vi "anna_results.vi"() -> ()   [LabVIEW 2009]
uses:
  <vilib>/Analysis/NI_AALPro.lvlib
panel:
  out "total spots":i32
  in  "add this file":bool
  out "All Files":path[](array[path])
  in  "clear xy":bool
  in  "store xy":bool
  out "XY Graph 2":cluster{"selected":dbl[], "selected":dbl[]}[](graph)
  in  "clear hist":bool
  in  "store hist":bool
  out "Histogram Graph 2":T1(graph)
  in  "export":bool
  in  "stop":bool
  in  "plot":bool
  out "selected":dbl[][](array[numeric])
  out "names":string[](array[string])
  out "XY Graph":cluster{"selected":dbl[], "selected":dbl[]}(graph)
  in  "plot y":u16(ring) items=["Spot No.", "plane", "Coordinates left", "Coordinates top", "Coordinates right", "Coordinates bottom", "TAC Window 1", "TAC Window 2", "Lifetime[ns] (sum)", "Lifetime[ns] (channel 1)", "Lifetime[ns] (channel 2)", "Lifetime[ns] (channel 3)", "tauerror (sum)", "tauerror (channel 1)", "tauerror (channel 2)", "tauerror (channel 3)", "F2-Value overall", "overall intensity (sum)", "overall intensity (channel 1)", "overall intensity (channel 2)", "overall intensity (channel 3)", "F2-Value TAC", "TAC intensity (sum)", "TAC intensity (channel 1)", "TAC intensity (channel 2)", "TAC intensity (channel 3)"]
  in  "plot x":u16(ring) items=["Spot No.", "plane", "Coordinates left", "Coordinates top", "Coordinates right", "Coordinates bottom", "TAC Window 1", "TAC Window 2", "Lifetime[ns] (sum)", "Lifetime[ns] (channel 1)", "Lifetime[ns] (channel 2)", "Lifetime[ns] (channel 3)", "tauerror (sum)", "tauerror (channel 1)", "tauerror (channel 2)", "tauerror (channel 3)", "F2-Value overall", "overall intensity (sum)", "overall intensity (channel 1)", "overall intensity (channel 2)", "overall intensity (channel 3)", "F2-Value TAC", "TAC intensity (sum)", "TAC intensity (channel 1)", "TAC intensity (channel 2)", "TAC intensity (channel 3)"]
  out "Histogram Graph":T2(graph)
  in  "# bins":i32
  in  "min":dbl format="%0.2f"
  in  "max":dbl format="%0.2f"
  in  "histogram":u16(ring) items=["Spot No.", "plane", "Coordinates left", "Coordinates top", "Coordinates right", "Coordinates bottom", "TAC Window 1", "TAC Window 2", "Lifetime[ns] (sum)", "Lifetime[ns] (channel 1)", "Lifetime[ns] (channel 2)", "Lifetime[ns] (channel 3)", "tauerror (sum)", "tauerror (channel 1)", "tauerror (channel 2)", "tauerror (channel 3)", "F2-Value overall", "overall intensity (sum)", "overall intensity (channel 1)", "overall intensity (channel 2)", "overall intensity (channel 3)", "F2-Value TAC", "TAC intensity (sum)", "TAC intensity (channel 1)", "TAC intensity (channel 2)", "TAC intensity (channel 3)"]
  in  "Selection":T3(array[cluster]) {"column" items=["Spot No.", "plane", "Coordinates left", "Coordinates top", "Coordinates right", "Coordinates bottom", "TAC Window 1", "TAC Window 2", "Lifetime[ns] (sum)", "Lifetime[ns] (channel 1)", "Lifetime[ns] (channel 2)", "Lifetime[ns] (channel 3)", "tauerror (sum)", "tauerror (channel 1)", "tauerror (channel 2)", "tauerror (channel 3)", "F2-Value overall", "overall intensity (sum)", "overall intensity (channel 1)", "overall intensity (channel 2)", "overall intensity (channel 3)", "F2-Value TAC", "TAC intensity (sum)", "TAC intensity (channel 1)", "TAC intensity (channel 2)", "TAC intensity (channel 3)"]}
  out "raw":dbl[][](array[numeric])
  in  "file (use dialog)":path
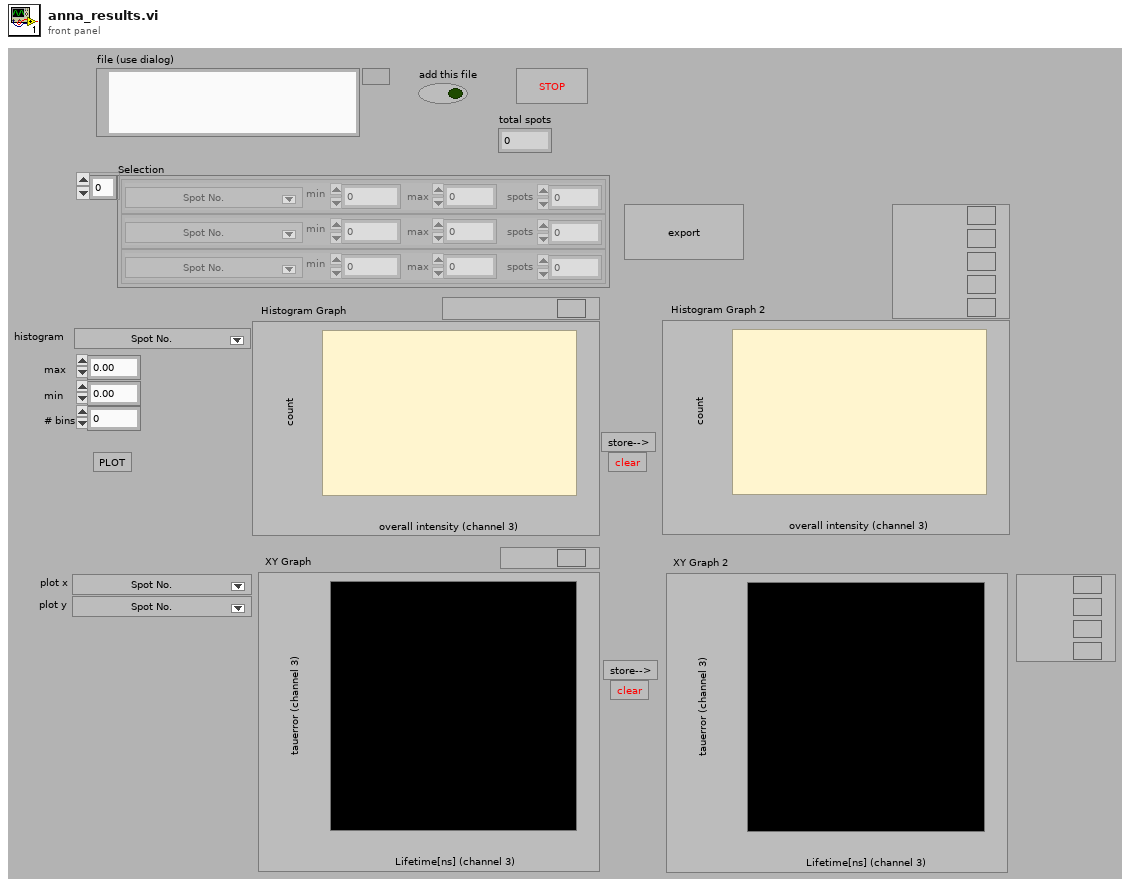
[diagram p1: front panel]
types:
  T1 = cluster{"X Values":dbl[], "Histogram: h(x)":i32[]}[]
  T2 = cluster{"X Values":dbl[], "Histogram: h(x)":i32[]}
  T3 = cluster{"column":u16, "min":dbl, "max":dbl, "spots ":i16}[]
  T4 = cluster{"column":u16, "min":dbl, "max":dbl, "spots ":i16}
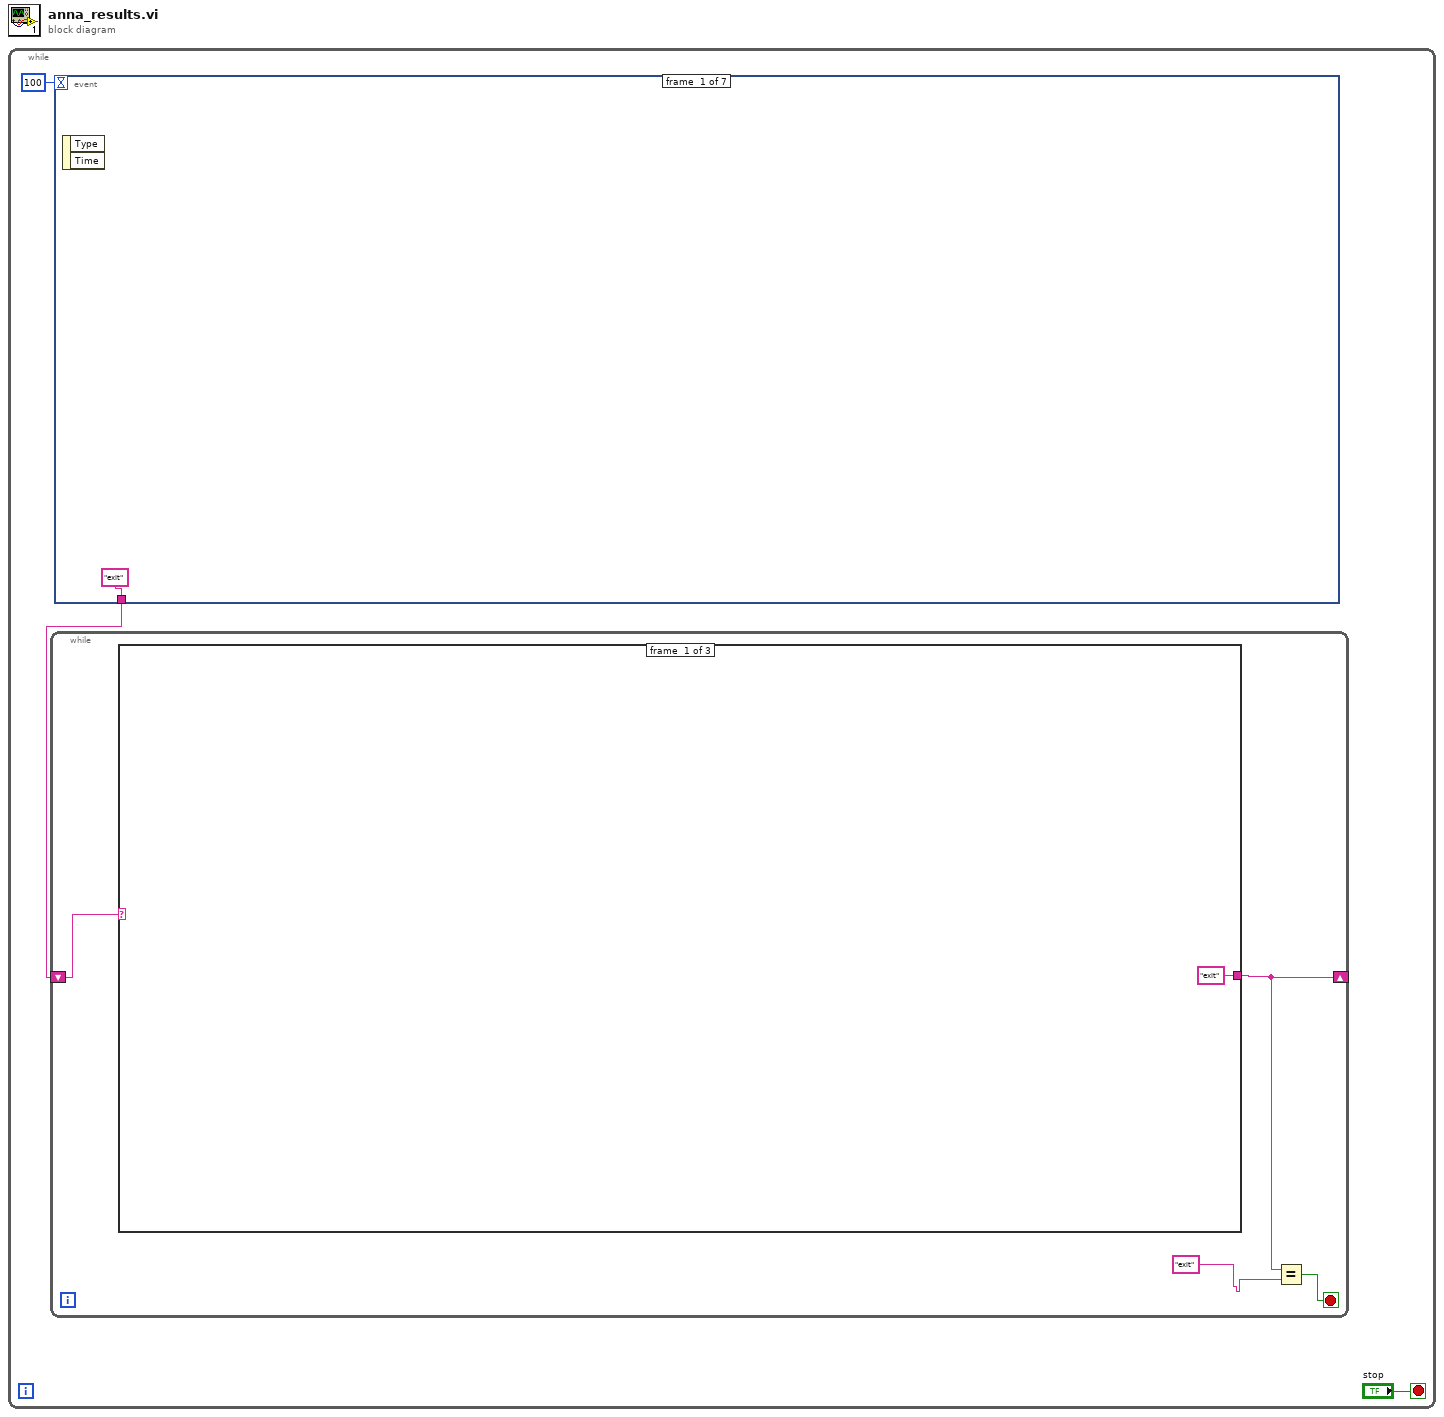
[diagram p0: block diagram]
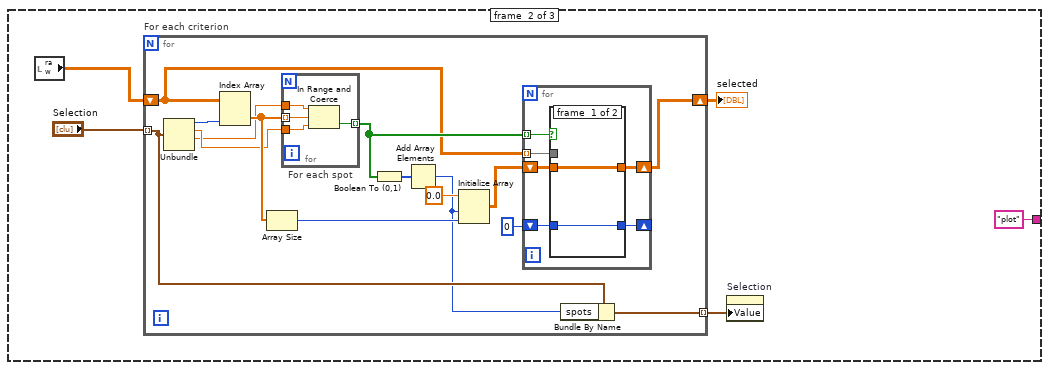
[diagram p2: hidden frame]
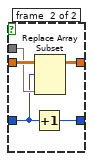
[diagram p3: hidden frame]
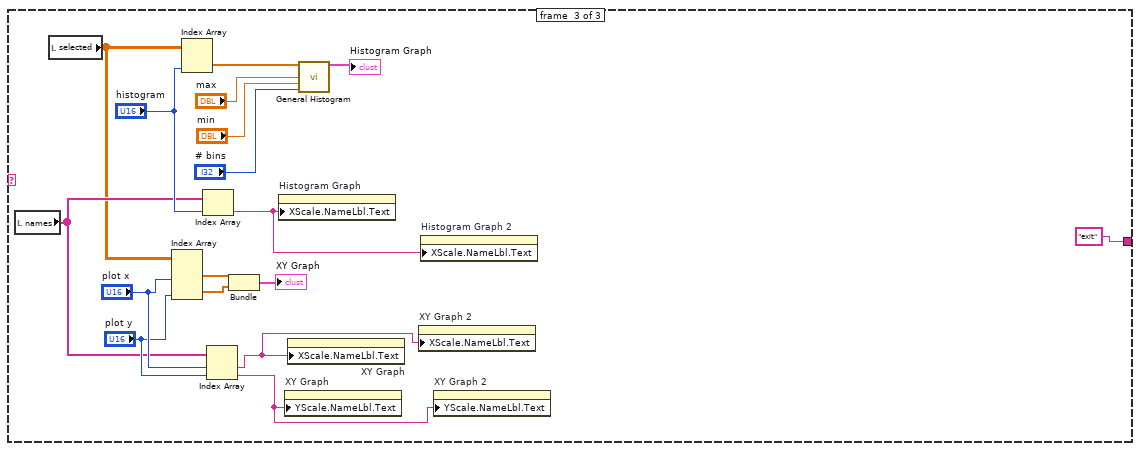
[diagram p4: hidden frame]
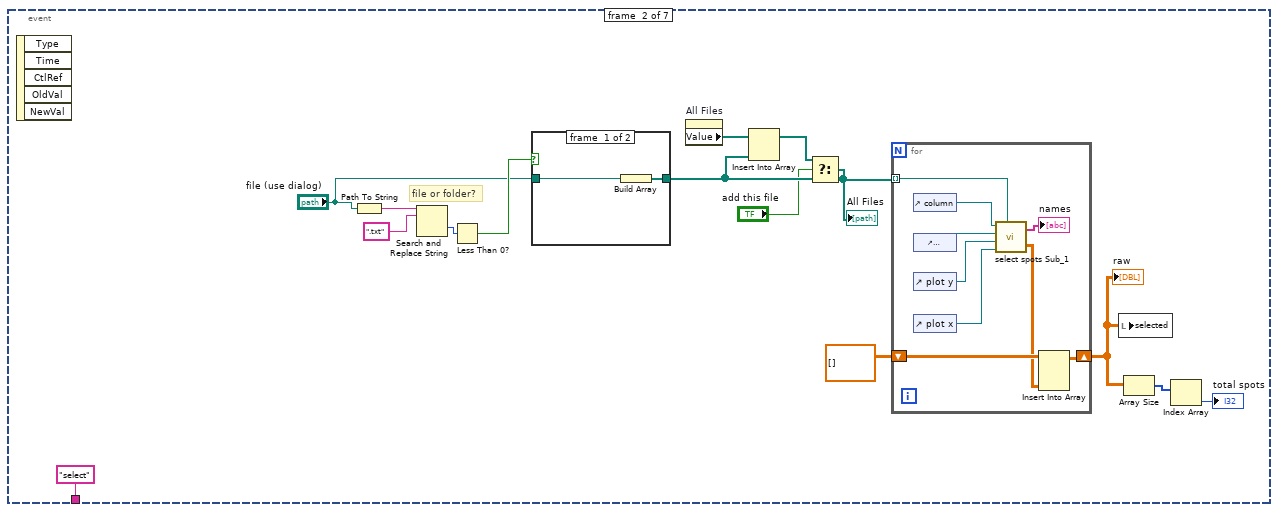
[diagram p5: hidden frame]
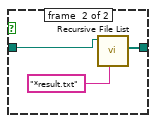
[diagram p6: hidden frame]
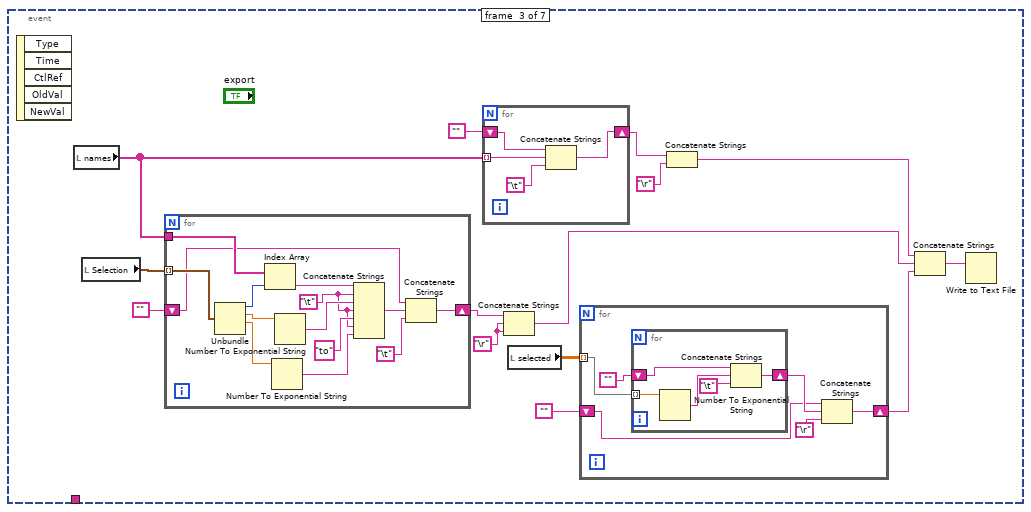
[diagram p7: hidden frame]
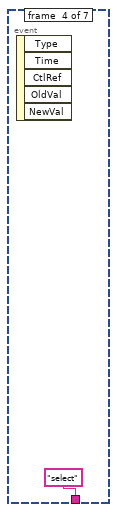
[diagram p8: hidden frame]
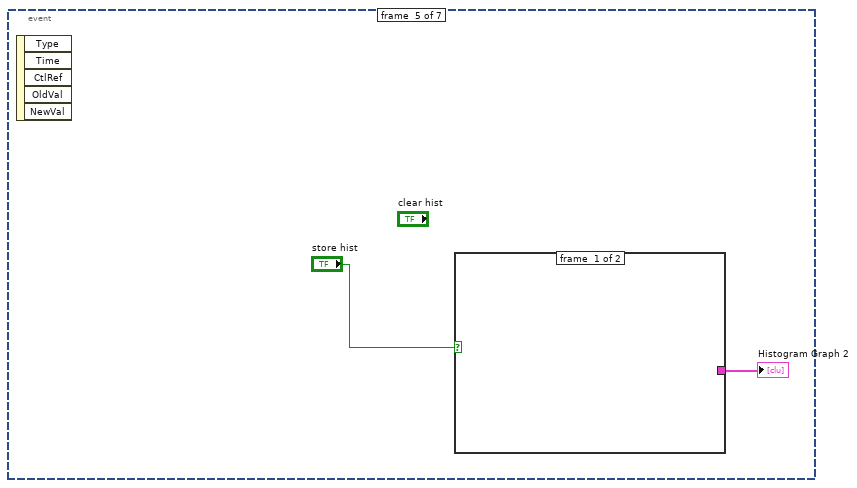
[diagram p9: hidden frame]
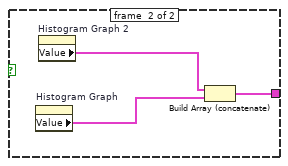
[diagram p10: hidden frame]
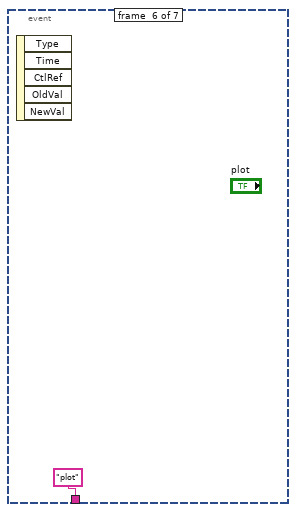
[diagram p11: hidden frame]
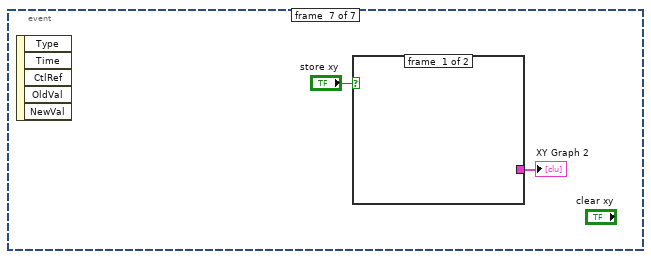
[diagram p12: hidden frame]
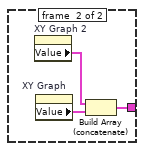
[diagram p13: hidden frame]
diagram:
  n1 = while {
    stop <- "stop" stop-if-true
    n2 = event shown="[1] \"file (use dialog)\": Value Change" {
      selector: _ -> [_ _ _ _ _ _ _]
      dyn-events: _ -> [_ _ _ _ _ _ _]
      timeout: 100 -> [_ _ _ _ _ _ _]
      tunnel: ["exit" "select" _ "select" _ "plot" _] -> w3
      event #0 {
        n3 = event-data() -> ()  [unwired: 1 in, 2 out]
      }
      event #1 {
        # "file or folder?"
        n4 = event-data() -> ()  [unwired: 1 in, 5 out]
        n5 = Path To String(path="file (use dialog)") -> (string=w76:string)
        n6 = Search and Replace String(input string=w76, search string=".txt") -> (offset past replacement=w74:i32)  [unwired: 6 in, 3 out]
        n7 = Less Than 0?(x=w74) -> (x < 0?=w73:bool)
        n8 = case shown="False" w73 {
          tunnel: [w79 w81] -> w69
          tunnel: "file (use dialog)" -> [w80 w83]
          frame #0 {
            n9 = Build Array(w80) -> (w79:path[])
          }
          frame #1 {
            n10 = call <vilib>:"Recursive File List.vi"("pattern"="*result.txt", "Folder Path"=w83) -> ("All Files in Dir"=w81:path[])  [unwired: 5 in, 4 out]
          }
        }
        n11 = property on="All Files" class="Arr (strict)"() -> ("Value"=w70:path[])  [unwired: 2 in, 2 out]
        n12 = Insert Into Array(array=w70, new element=w69) -> (w68:path[])  [unwired: 1 in]
        n13 = Select(t=w68, s="add this file", f=w69) -> (s? t:f=w71:path[])
        "All Files" <- w71
        n14 = for {
          tunnel: w71 -> [w87] mode=indexing
          shift-right: [w84] -> w66
          shift-left: dbl[][] [] ("Array") -> [w86]
          n15 = control-ref of="column"() -> (w92:refnum<vi>)
          n16 = control-ref of="histogram"() -> (w91:refnum<vi>)
          n17 = control-ref of="plot y"() -> (w90:refnum<vi>)
          n18 = control-ref of="plot x"() -> (w89:refnum<vi>)
          n19 = call "select spots Sub_1.vi"("Ring Refnum"=w92, "Ring Refnum 2"=w91, "Ring Refnum 3"=w90, "Ring Refnum 4"=w89, "file (use dialog)"=w87) -> ("names"=→"names":string[], "Array"=w85:dbl[][])
          n20 = Insert Into Array(array=w86, new element=w85) -> (w84:dbl[][])  [unwired: 2 in]
        }
        "raw" <- w66
        n21 = local write "selected"(w66) -> ()
        n22 = Array Size(array=w66) -> (size(s)=w65:i32[])
        n23 = Index Array(array=w65) -> (element=→"total spots":i32)  [unwired: 1 in]
      }
      event #2 {
        w96 = "\r"
        n24 = event-data() -> ()  [unwired: 1 in, 5 out]
        n25 = local read "names"() -> (w101:string[])
        n26 = local read "Selection"() -> (w102:T3)
        n27 = for {
          tunnel: w102 -> [w119] mode=indexing
          tunnel: w101 -> [w120]
          shift-right: [w111] -> w99
          shift-left: "" -> [w110]
          w107 = "\t"
          n28 = Unbundle(w119) -> ("column"=w118:u16, "min"=w117:dbl, "max"=w116:dbl)  [unwired: 1 out]
          n29 = Index Array(array=w120, index=w118) -> (element=w115:string)
          n30 = Number To Exponential String(number=w116) -> (E-format string=w108:string)  [unwired: 3 in]
          n31 = Number To Exponential String(number=w117) -> (E-format string=w114:string)  [unwired: 3 in]
          n32 = Concatenate Strings(w115, w107, w114, w107, "to" ("string"), w107, w108) -> (w113:string)
          n33 = Concatenate Strings(w110, w113, "\t") -> (w111:string)
        }
        n34 = for {
          tunnel: w101 -> [w135] mode=indexing
          shift-right: [w133] -> w105
          shift-left: "" -> [w132]
          n35 = Concatenate Strings(w132, w135, "\t") -> (w133:string)
        }
        n36 = Concatenate Strings(w99, w96, w96) -> (w97:string)
        n37 = local read "selected"() -> (w94:dbl[][])
        n38 = for {
          tunnel: w94 -> [w126] mode=indexing
          shift-right: [w122] -> w98
          shift-left: "" -> [w121]
          n39 = for {
            tunnel: w126 -> [w131] mode=indexing
            shift-right: [w127] -> w124
            shift-left: "" -> [w129]
            n40 = Number To Exponential String(number=w131) -> (E-format string=w128:string)  [unwired: 3 in]
            n41 = Concatenate Strings(w129, w128, "\t") -> (w127:string)
          }
          n42 = Concatenate Strings(w121, w124, "\r") -> (w122:string)
        }
        n43 = Concatenate Strings(w105, "\r") -> (w103:string)
        n44 = Concatenate Strings(w103, w97, w98) -> (w95:string)
        n45 = Write to Text File(text=w95) -> ()  [unwired: 3 in, 3 out]
      }
      event #3 {
        n46 = event-data() -> ()  [unwired: 1 in, 5 out]
      }
      event #4 {
        n47 = event-data() -> ()  [unwired: 1 in, 5 out]
        n48 = case shown="True" "store hist" {
          tunnel: [_ w139] -> w138
          frame #0 {
          }
          frame #1 {
            n49 = property on="Histogram Graph" class="XYGraph (strict)"() -> ("Value"=w140:T2)  [unwired: 2 in, 2 out]
            n50 = property on="Histogram Graph 2" class="XYGraph (strict)"() -> ("Value"=w141:T1)  [unwired: 2 in, 2 out]
            n51 = Build Array (concatenate)(w141, w140) -> (w139:T1)
          }
        }
        "Histogram Graph 2" <- w138
      }
      event #5 {
        n52 = event-data() -> ()  [unwired: 1 in, 5 out]
      }
      event #6 {
        n53 = event-data() -> ()  [unwired: 1 in, 5 out]
        n54 = case shown="True" "store xy" {
          tunnel: [_ w145] -> w143
          frame #0 {
          }
          frame #1 {
            n55 = property on="XY Graph 2" class="XYGraph (strict)"() -> ("Value"=w147:cluster{"selected":dbl[], "selected":dbl[]}[])  [unwired: 2 in, 2 out]
            n56 = property on="XY Graph" class="XYGraph (strict)"() -> ("Value"=w146:cluster{"selected":dbl[], "selected":dbl[]})  [unwired: 2 in, 2 out]
            n57 = Build Array (concatenate)(w147, w146) -> (w145:cluster{"selected":dbl[], "selected":dbl[]}[])
          }
        }
        "XY Graph 2" <- w143
      }
    }
    n58 = while {
      shift-right: [w5] -> _
      shift-left: w3 -> [w4]
      stop <- w7 stop-if-true
      n59 = case shown="\"select\"" w4 {
        tunnel: ["exit" "plot" "exit"] -> w5
        frame #0 {
        }
        frame #1 {
          n60 = local read "raw"() -> (w11:dbl[][])
          n61 = for "For each criterion" {
            shift-right: [w22] -> w10
            shift-left: w11 -> [w21]
            tunnel: "Selection" -> [w16] mode=indexing
            tunnel: [w14] -> w12 mode=indexing
            n62 = Unbundle(w16) -> ("column"=w19:u16, "min"=w18:dbl, "max"=w17:dbl)  [unwired: 1 out]
            n63 = Index Array(array=w21, index (col)=w19) -> (element=w20:dbl[])  [unwired: 1 in]
            n64 = Array Size(array=w20) -> (size(s)=w25:i32)
            n65 = for "For each spot" {
              tunnel: w20 -> [w43] mode=indexing
              tunnel: w17 -> [w45]
              tunnel: w18 -> [w44]
              tunnel: [w42] -> w28 mode=indexing
              n66 = In Range and Coerce(upper limit=w45, x=w43, lower limit=w44) -> (In Range?=w42:bool)  [unwired: 1 out]
            }
            n67 = Boolean To (0,1)(Boolean=w28) -> (0, 1=w27:i16[])
            n68 = Add Array Elements(numeric array=w27) -> (sum=w15:i16)
            n69 = Initialize Array(0.0, w15, w25) -> (w24:dbl[][])
            n70 = for {
              tunnel: w28 -> [w31] mode=indexing
              tunnel: w21 -> [w33] mode=indexing
              shift-right: [w32] -> w22
              shift-left: w24 -> [w34]
              shift-right: [w29] -> _
              shift-left: 0 -> [w30]
              n71 = case shown="True" w31 {
                tunnel: w34 -> [w36 w41]
                tunnel: w33 -> [_ w40]
                tunnel: [w36 w39] -> w32
                tunnel: w30 -> [w35 w37]
                tunnel: [w35 w38] -> w29
                frame #0 {
                }
                frame #1 {
                  n72 = Increment(x=w37) -> (x+1=w38:i32)
                  n73 = Replace Array Subset(array=w41, new element=w40, index (row)=w37) -> (w39:dbl[][])  [unwired: 1 in]
                }
              }
            }
            n74 = Bundle By Name(cluster=w16, "spots"=w15) -> (w14:T4)
          }
          "selected" <- w10
          n75 = property on="Selection" class="Arr (strict)"("Value"=w12) -> ()  [unwired: 2 in, 2 out]
        }
        frame #2 {
          n76 = local read "names"() -> (w53:string[])
          n77 = local read "selected"() -> (w52:dbl[][])
          n78 = Index Array(array=w52, index (col) #1="plot x", index (col) #2="plot y") -> (element #1=w58:dbl[], element #2=w57:dbl[])  [unwired: 2 in]
          n79 = Index Array(array=w52, index (col)="histogram") -> (element=w62:dbl[])  [unwired: 1 in]
          n80 = Index Array(array=w53, index="histogram") -> (element=w48:string)
          n81 = Index Array(array=w53, index #1="plot x", index #2="plot y") -> (element #1=w47:string, element #2=w46:string)
          n82 = Bundle("selected"=w58, "selected"=w57) -> (→"XY Graph":cluster{"selected":dbl[], "selected":dbl[]})  [unwired: 1 in]
          n83 = property on="Histogram Graph" class="XYGraph (strict)"("XScale.NameLbl.Text"=w48) -> ()  [unwired: 2 in, 2 out]
          n84 = property on="XY Graph" class="XYGraph (strict)"("YScale.NameLbl.Text"=w46) -> ()  [unwired: 2 in, 2 out]
          n85 = property on="XY Graph" class="XYGraph (strict)"("XScale.NameLbl.Text"=w47) -> ()  [unwired: 2 in, 2 out]
          n86 = call <vilib>:"General Histogram.vi"("X"=w62, "max"="max", "min"="min", "# bins"="# bins") -> ("Histogram Graph"=→"Histogram Graph":T2)  [unwired: 7 in, 4 out]
          n87 = property on="XY Graph 2" class="XYGraph (strict)"("XScale.NameLbl.Text"=w47) -> ()  [unwired: 2 in, 2 out]
          n88 = property on="Histogram Graph 2" class="XYGraph (strict)"("XScale.NameLbl.Text"=w48) -> ()  [unwired: 2 in, 2 out]
          n89 = property on="XY Graph 2" class="XYGraph (strict)"("YScale.NameLbl.Text"=w46) -> ()  [unwired: 2 in, 2 out]
        }
      }
      n90 = Equal?(x=w5, y="exit") -> (x = y?=w7:bool)
    }
  }
